vi "Display Console View.vi"(8 "error in (no error)":errorcluster, 11 "View Model":T2) -> (0 "error out":errorcluster)   [LabVIEW 2017]
doc: "The interface where a user receives status updates from the controller.\n[Covers: UI3]"
uses:
  View Model/Controls/View Model.ctl
  View Model/Controls/Shared Model.ctl
  Error Handler/Controls/Error Model.ctl
  Error Handler/Controls/Error Data.ctl
  Error Handler/Controls/Error Level.ctl
  Configuration/Controls/Config Model.ctl
  Configuration/Controls/Config Data Record.ctl
  Configuration/Controls/Config Command.ctl
  Controller/Controls/Control Model.ctl
  Controller/Controls/Elevator Location.ctl
  Controller/Controls/Elevator Status.ctl
  Controller/Controls/Control Event.ctl
  Controller/Controls/Control CMD.ctl
panel:
  out "Timing":dbl
  out "Elevator Location":T1
  out "Emergency":bool
  out "Door Open":bool
  out "Down":bool
  out "Up":bool
  # "Elevator Directions"
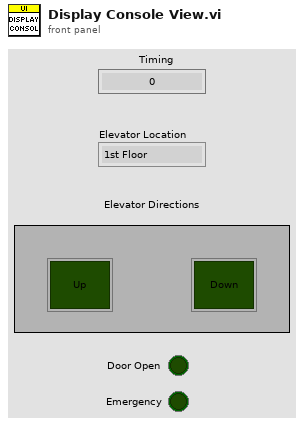
[diagram p1: front panel]
types:
  T1 = typedef "Elevator Location.ctl" = enum16{"1st Floor", "2nd Floor", "3rd Floor", "4th Floor"}
  T2 = typedef "View Model.ctl" = cluster{"Shared Model":T3, "Error Model":T4, "Config Model":T5, "Control Model":T6}
  T3 = typedef "Shared Model.ctl" = cluster{"Stop":refnum<user-event>, "Stop DVR":refnum<data-value>}
  T4 = typedef "Error Model.ctl" = cluster{"Error":refnum<user-event>}
  T5 = typedef "Config Model.ctl" = cluster{"Data DVR":refnum<data-value>, "Config CMD":refnum<user-event>}
  T6 = typedef "Control Model.ctl" = cluster{"Location Change":refnum<user-event>, "Location DVR":refnum<data-value>, "Elapsed Time DVR":refnum<data-value>, "Direction Change":refnum<user-event>, "Door Posit Change":refnum<user-event>, "Emergency Change":refnum<user-event>, "Status Change":refnum<user-event>, "Status DVR":refnum<data-value>, "Command":refnum<user-event>}
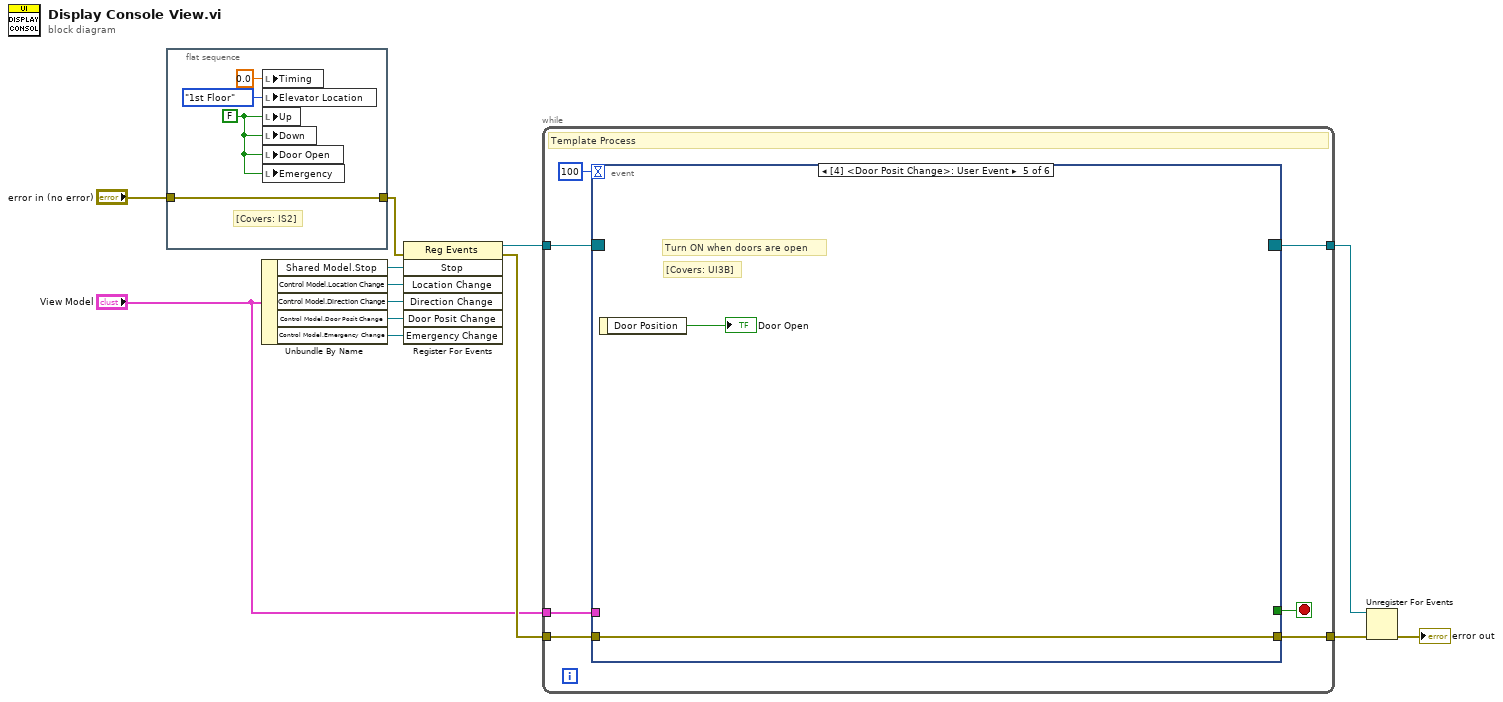
[diagram p0: block diagram]
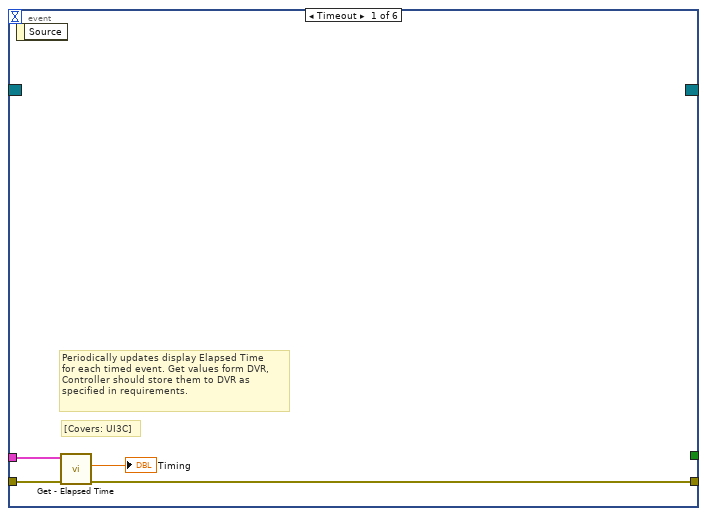
[diagram p2: hidden frame]
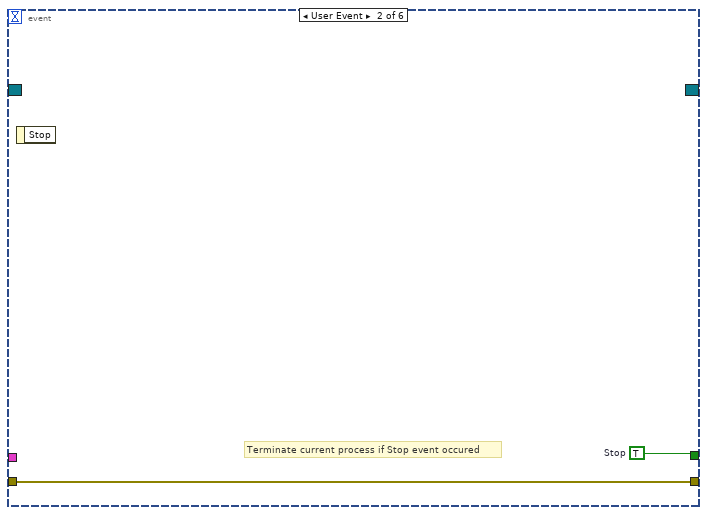
[diagram p3: hidden frame]
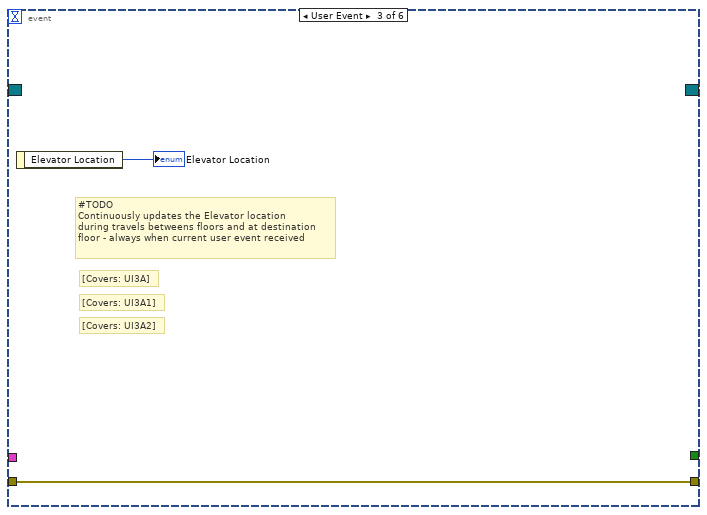
[diagram p4: hidden frame]
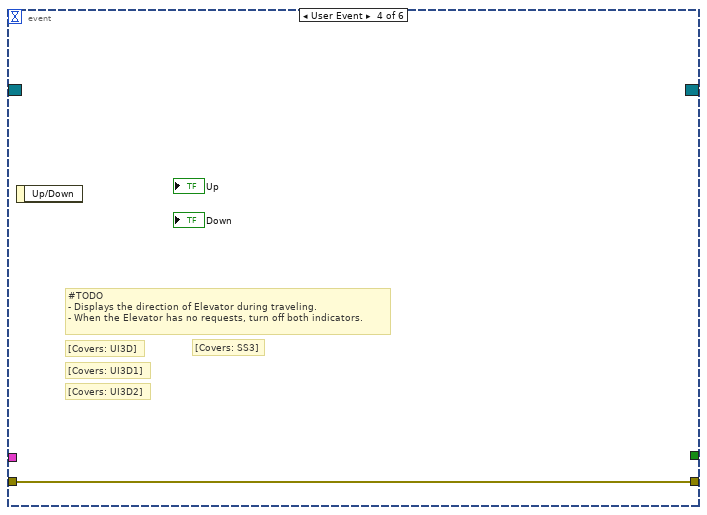
[diagram p5: hidden frame]
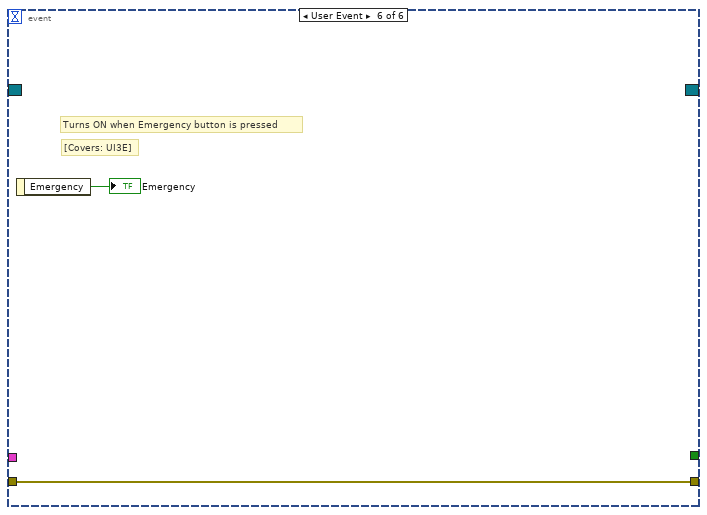
[diagram p6: hidden frame]
diagram:
  n1 = flat-sequence {
    tunnel: "error in (no error)" -> [w14]
    tunnel: [w14] -> w1
    frame #0 {
      w17 = FALSE ("Up")
      # "[Covers: IS2]"
      n2 = local write "Timing"(0.0 ("Timing")) -> ()
      n3 = local write "Elevator Location"(Elevator_Location."1st Floor" ("Elevator Location")) -> ()
      n4 = local write "Up"(w17) -> ()
      n5 = local write "Down"(w17) -> ()
      n6 = local write "Door Open"(w17) -> ()
      n7 = local write "Emergency"(w17) -> ()
    }
  }
  n8 = Unbundle By Name("View Model") -> ("Shared Model.Stop"=w13:refnum<user-event>, "Control Model.Location Change"=w7:refnum<user-event>, "Control Model.Direction Change"=w3:refnum<user-event>, "Control Model.Door Posit Change"=w4:refnum<user-event>, "Control Model.Emergency Change"=w5:refnum<user-event>)
  n9 = register-events(error in=w1, w13, w7, w3, w4, w5) -> (reference out=w12:refnum<event-registration>, error out=w11:errorcluster)  [unwired: 1 in]
  n10 = while {
    tunnel: w12 -> [w24]
    tunnel: w11 -> [w23]
    tunnel: [w22] -> w9
    tunnel: [w20] -> w10
    tunnel: "View Model" -> [w18]
    stop <- w21 stop-if-true
    # "Template Process"
    n11 = event shown="[4] <Door Posit Change>: User Event" {
      selector: w24 -> [_ _ _ _ _ _]
      dyn-events: [_ _ _ _ _ _] -> w20
      timeout: 100 -> [_ _ _ _ _ _]
      tunnel: w23 -> [w28 w30 w32 w33 w35 w37]
      tunnel: [w26 w30 w32 w33 w35 w37] -> w22
      tunnel: [_ w29 _ _ _ _] -> w21
      tunnel: w18 -> [w27 _ _ _ _ _]
      event Timeout {
        # "[Covers: UI3C]"
        # "Periodically updates display Elapsed Time\nfor each timed event. Get values form DVR,\nController should store them to DVR as \nspecified in requirements."
        n12 = event-data() -> ()  [unwired: 1 in, 1 out]
        n13 = call "Get - Elapsed Time.vi"("error in (no error)"=w28, "View Model"=w27) -> ("error out"=w26:errorcluster, "Elapsed Time"=→"Timing":dbl)  [unwired: 7 in, 1 out]
      }
      event User Event {
        w29 = TRUE  # Stop
        # "Terminate current process if Stop event occured"
        n14 = event-data() -> ()  [unwired: 1 in, 1 out]
      }
      event User Event {
        # "[Covers: UI3A2]"
        # "[Covers: UI3A1]"
        # "[Covers: UI3A]"
        # "#TODO\nContinuously updates the Elevator location\nduring travels betweens floors and at destination\nfloor - always when current user event received"
        n15 = event-data() -> ("Elevator Location"=→"Elevator Location":T1)  [unwired: 1 in]
      }
      event User Event {
        # "[Covers: SS3]"
        # "[Covers: UI3D2]"
        # "[Covers: UI3D1]"
        # "[Covers: UI3D]"
        # "#TODO\n- Displays the direction of Elevator during traveling.\n- When the Elevator has no requests, turn off both indicators."
        n16 = event-data() -> ()  [unwired: 1 in, 1 out]
      }
      event User Event {
        # "[Covers: UI3B]"
        # "Turn ON when doors are open"
        n17 = event-data() -> ("Door Position"=→"Door Open":bool)  [unwired: 1 in]
      }
      event User Event {
        # "[Covers: UI3E]"
        # "Turns ON when Emergency button is pressed"
        n18 = event-data() -> ("Emergency"=→"Emergency":bool)  [unwired: 1 in]
      }
    }
  }
  n19 = Unregister For Events(event registration refnum=w10, error in=w9) -> (error out=→"error out":errorcluster)
